vi "AreaAroundSelNode.vi"(6 "Distance":i16=10, 11 "Master Bounds Rect":T1) -> (3 "Bounds+Distance":T1)   [LabVIEW 2014]
uses:
  <vilib>/Utility/miscctls.llb/LVRectTypeDef.ctl
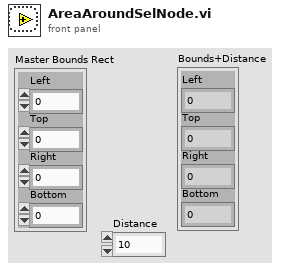
[diagram p1: front panel]
types:
  T1 = typedef "LVRectTypeDef.ctl" = cluster{"Left":i16, "Top":i16, "Right":i16, "Bottom":i16}
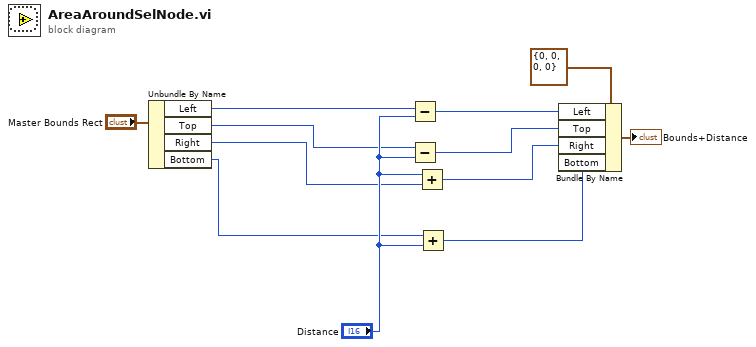
[diagram p0: block diagram]
diagram:
  n1 = Unbundle By Name("Master Bounds Rect") -> ("Left"=w10:i16, "Top"=w9:i16, "Right"=w8:i16, "Bottom"=w7:i16)
  n2 = Subtract(x=w10, y="Distance") -> (x-y=w5:i16)
  n3 = Subtract(x=w9, y="Distance") -> (x-y=w4:i16)
  n4 = Add(x="Distance", y=w8) -> (x+y=w3:i16)
  n5 = Add(x=w7, y="Distance") -> (x+y=w2:i16)
  n6 = Bundle By Name(cluster=T1 {"Left"=0, "Top"=0, "Right"=0, "Bottom"=0} ("Master Bounds Rect"), "Left"=w5, "Top"=w4, "Right"=w3, "Bottom"=w2) -> (→"Bounds+Distance":T1)
